vi "일정거리를 계속해서 유지하는 로봇.vi"() -> ()   [LabVIEW 2010]
uses:
  <vilib>/NXT/Subs/MotorOutput.ctl
  <vilib>/NXT/Block Support/NXT_InputPort.ctl
  <vilib>/NXT/Dual Mode Library/Motors/MotorOn.vi
panel:
  in  "target distance":dbl(slide) scale=0.0..10.0
  out "distance":dbl(slide) scale=0.0..10.0
  out "Distance (cm)":i16
  in  "stop":bool
  in  "Power (75)":i32=75
  in  "Output Port (All Ports)":T1=3 items=["Port A", "Port B", "Port C", "All Ports"]
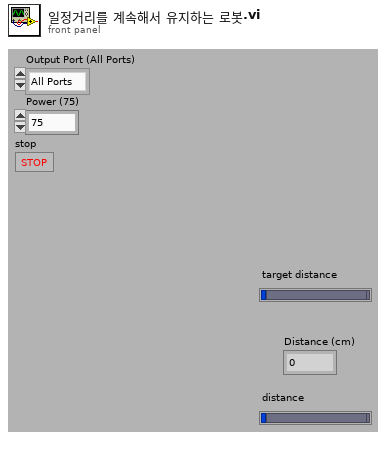
[diagram p1: front panel]
types:
  T1 = typedef "MotorOutput.ctl" = u8
  T2 = typedef "NXT_InputPort.ctl" = u8
  T3 = typedef "LVHSConnector.ctl" = cluster{"error":errorcluster, "address":string, "NXT #":i32, "Show Error":bool, "Connection":u16}
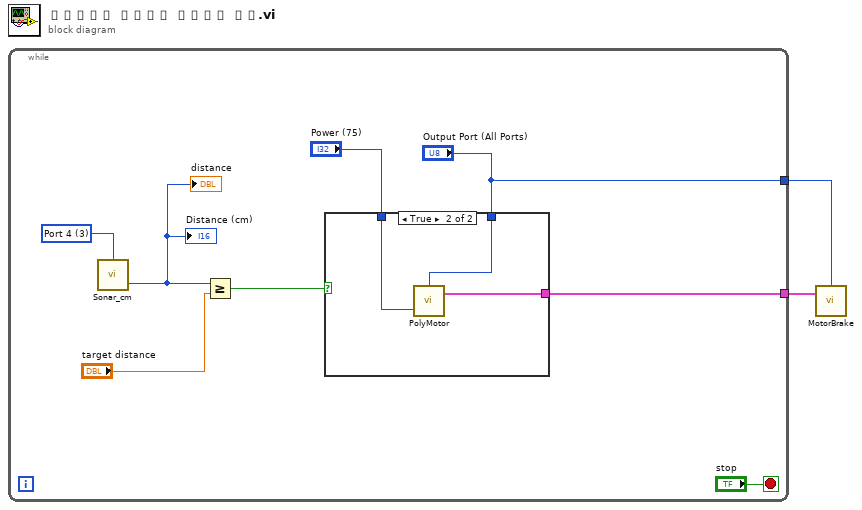
[diagram p0: block diagram]
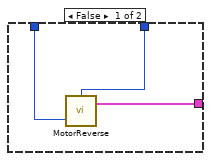
[diagram p2: hidden frame]
diagram:
  n1 = while {
    tunnel: ["Output Port (All Ports)"] -> w2
    tunnel: [w4] -> w1
    stop <- "stop" stop-if-true
    w6 = T2 3 items=["Port 1", "Port 2", "Port 3", "Port 4"] ("Port (Port 4)")
    n2 = call <vilib>:"Sonar_cm.vi"("Port (Port 4)"=w6) -> ("Distance (cm)"=w5:i16)  [unwired: 2 in, 1 out]
    "Distance (cm)" <- w5
    "distance" <- w5
    n3 = Greater Or Equal?(x=w5, y="target distance") -> (x >= y?=w10:bool)
    n4 = case shown="True" w10 {
      tunnel: [w13 w14] -> w4
      tunnel: "Output Port (All Ports)" -> [w12 w16]
      tunnel: "Power (75)" -> [w11 w15]
      frame False {
        n5 = call <vilib>:"MotorReverse.vi"("Power (75)"=w11, "Output Port (All Ports)"=w12) -> ("NXT"=w13:T3)  [unwired: 2 in]
      }
      frame True {
        n6 = call-poly <vilib>:"PolyMotor.vi"("Power (75)"=w15, "Output Port (All Ports)"=w16) -> ("NXT"=w14:T3)  [unwired: 2 in]
      }
    }
  }
  n7 = call <vilib>:"MotorBrake.vi"("NXT"=w1, "Port (All Ports)"=w2) -> ()  [unwired: 2 in, 1 out]
